vi "Fetch Digital Waveform.vi"(8 "error in (no error)":errorcluster, 10 "Timeout (10000 ms)":u32=10000, 11 "VISA resource name":refnum<visa-resource-name>) -> (0 "error out":errorcluster, 2 "Digital Waveform Graph":digitalwaveform(graph), 3 "VISA resource name out":refnum<visa-resource-name>)   [LabVIEW 2023, in "RIGOL DS1054Z Driver.lvlib"]
doc: "Returns the waveform the oscilloscope acquired for the digital channel. \n\n<B>Note:</B>\n Use this VI only with other low-level VIs."
uses:
  <instrlib>/RIGOL-DS1054Z-LabVIEW/RIGOL DS1054Z Driver.lvlib
  <vilib>/Waveform/DWDTOps.llb/DWDT Binary U32 to Digital.vi
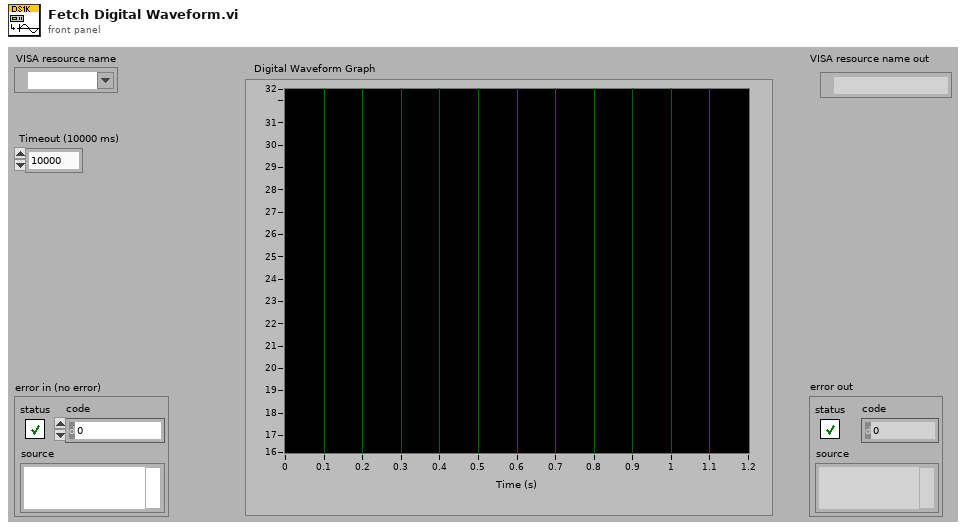
[diagram p1: front panel]
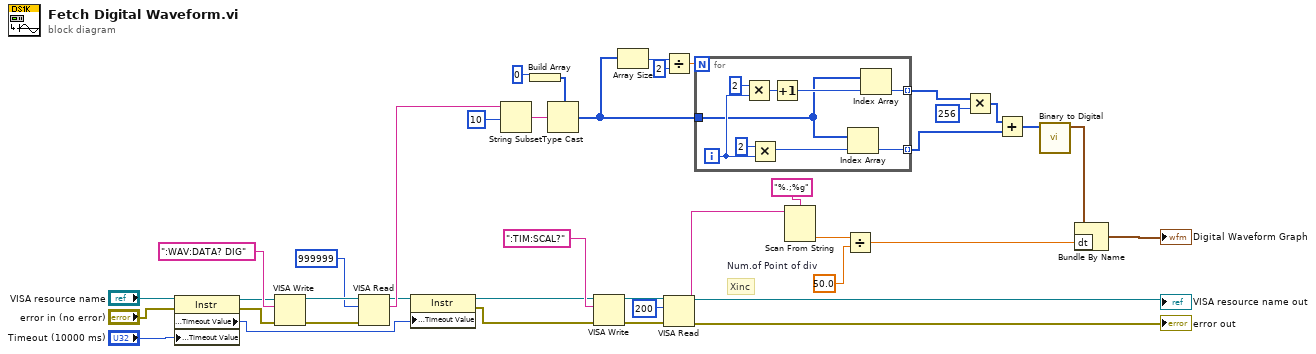
[diagram p0: block diagram]
diagram:
  w9 = 50.0  # Num.of Point of div
  # "Xinc"
  n1 = property class="Instr"(reference="VISA resource name", error in="error in (no error)", "General Settings:Timeout Value"="Timeout (10000 ms)") -> (reference out=w22:refnum<visa-resource-name>, error out=w20:errorcluster, "General Settings:Timeout Value"=w17:u32)
  n2 = VISA Write(VISA resource name=w22, write buffer=":WAV:DATA? DIG" ("写入缓冲区"), error in (no error)=w20) -> (VISA resource name out=w33:refnum<visa-resource-name>, error out=w26:errorcluster)  [unwired: 1 out]
  n3 = VISA Read(VISA resource name=w33, byte count=u32 999999 ("字节总数"), error in (no error)=w26) -> (VISA resource name out=w19:refnum<visa-resource-name>, read buffer=w29:string)  [unwired: 2 out]
  n4 = property class="Instr"(reference=w19, "General Settings:Timeout Value"=w17) -> (reference out=w8:refnum<visa-resource-name>, error out=w7:errorcluster)  [unwired: 1 in]
  n5 = String Subset(string=w29, offset (0)=10 ("偏移量(0)")) -> (substring=w27:string)  [unwired: 1 out]
  n6 = Build Array(u8 0) -> (w30:u8[])
  n7 = Type Cast(type=w30, x=w27) -> (*(type *) &x=w34:u8[])
  n8 = VISA Write(VISA resource name=w8, write buffer=":TIM:SCAL?", error in (no error)=w7) -> (VISA resource name out=w15:refnum<visa-resource-name>, error out=w14:errorcluster)  [unwired: 1 out]
  n9 = Array Size(array=w34) -> (size(s)=w35:i32)
  n10 = Divide(x=w35, y=2) -> (x/y=w36:dbl)
  n11 = VISA Read(VISA resource name=w15, byte count=u32 200, error in (no error)=w14) -> (VISA resource name out=→"VISA resource name out":refnum<visa-resource-name>, read buffer=w11:string, error out=→"error out":errorcluster)  [unwired: 1 out]
  n12 = for {
    N: w36 -> [_]
    tunnel: w34 -> [w42]
    tunnel: [w47] -> w25 mode=indexing
    tunnel: [w41] -> w38 mode=indexing
    i -> [w45]
    n13 = Multiply(x=2, y=w45) -> (x*y=w44:i32)
    n14 = Multiply(x=2, y=w45) -> (x*y=w48:i32)
    n15 = Increment(x=w44) -> (x+1=w43:i32)
    n16 = Index Array(array=w42, index=w48) -> (element=w47:u8)
    n17 = Index Array(array=w42, index=w43) -> (element=w41:u8)
  }
  n18 = Scan From String(format string="%.;%g", input string=w11) -> (output 1=w10:dbl)  [unwired: 2 in, 4 out]
  n19 = Divide(x=w10, y=w9) -> (x/y=w2:dbl)
  n20 = Multiply(x=w38, y=256) -> (x*y=w40:i32[])
  n21 = Add(x=w40, y=w25) -> (x+y=w1:i32[])
  n22 = call-poly <vilib>:"Binary to Digital.vi"("binary array"=w1) -> ("digital waveform"=w4:digitalwaveform)  [unwired: 3 in, 7 out]
  n23 = Bundle By Name(cluster=w4, "dt"=w2) -> (→"Digital Waveform Graph":digitalwaveform)
